vi "MaxVelGivenRadius.vi"() -> ()   [LabVIEW 2017]
panel:
  out "output variable":dbl
  in  "Vmax":dbl
  in  "Trackwidth":dbl
  in  "Radius":dbl
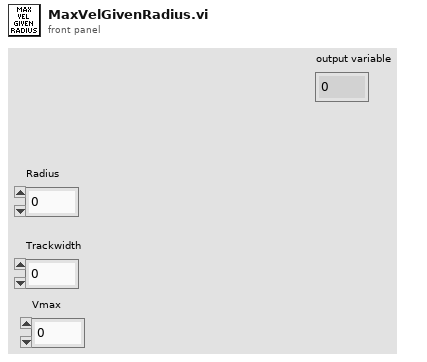
[diagram p1: front panel]
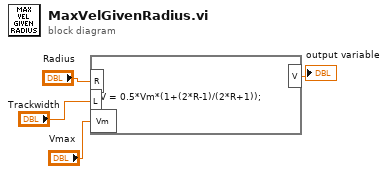
[diagram p0: block diagram]
diagram:
  n1 = formula code="V = 0.5*Vm*(1+(2*R-1)/(2*R+1));"("R"="Radius", "L"="Trackwidth", "Vm"="Vmax") -> ("V"=→"output variable":dbl)
